vi "new_issue_full.vi"(11 "issueInfo":T1) -> (3 "issue_class out":refnum<class "issue_class.lvclass">)   [LabVIEW 2024, in "issue_class.lvclass"]
uses:
  issue_class.lvclass
  comic_class/issueInfo--cluster.ctl
  comic_class/creator--cluster.ctl
  comic_class/character--cluster.ctl
  comic_class/team--cluster.ctl
  comic_class/location--cluster.ctl
  comic_class/concept--cluster.ctl
  comic_class/thing--cluster.ctl
  comic_class/storyArc--cluster.ctl
  issue_class.lvclass/issue_class.ctl
  comic_class/comic_class.lvclass
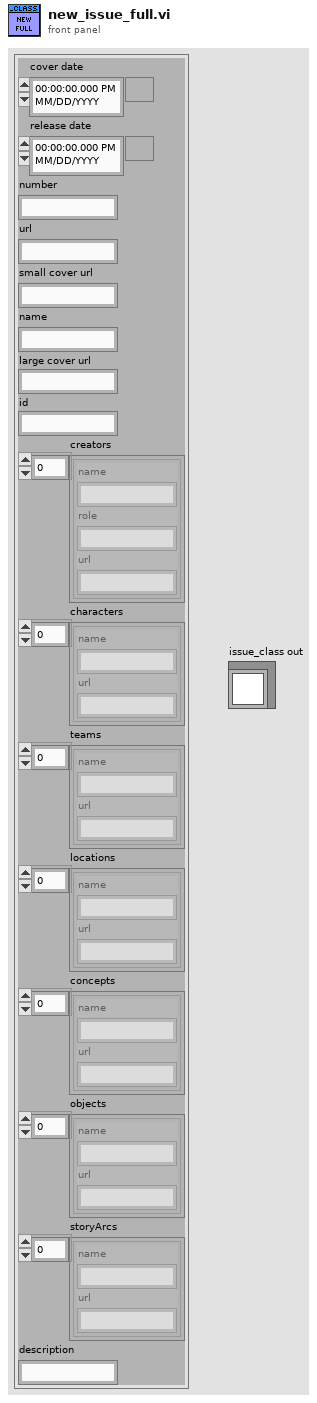
[diagram p1: front panel]
types:
  T1 = typedef "comic_class.lvclass/issueInfo--cluster.ctl" = cluster{"cover date":timestamp, "release date":timestamp, "number":string, "url":string, "small cover url":string, "name":string, "large cover url":string, "id":string, "creators":T2[], "characters":T3[], "teams":T4[], "locations":T5[], "concepts":T6[], "objects":T7[], "storyArcs":T8[], "description":string}
  T2 = typedef "comic_class.lvclass/creator--cluster.ctl" = cluster{"name":string, "role":string, "url":string}
  T3 = typedef "comic_class.lvclass/character--cluster.ctl" = cluster{"name":string, "url":string}
  T4 = typedef "comic_class.lvclass/team--cluster.ctl" = cluster{"name":string, "url":string}
  T5 = typedef "comic_class.lvclass/location--cluster.ctl" = cluster{"name":string, "url":string}
  T6 = typedef "comic_class.lvclass/concept--cluster.ctl" = cluster{"name":string, "url":string}
  T7 = typedef "comic_class.lvclass/thing--cluster.ctl" = cluster{"name":string, "url":string}
  T8 = typedef "comic_class.lvclass/storyArc--cluster.ctl" = cluster{"name":string, "url":string}
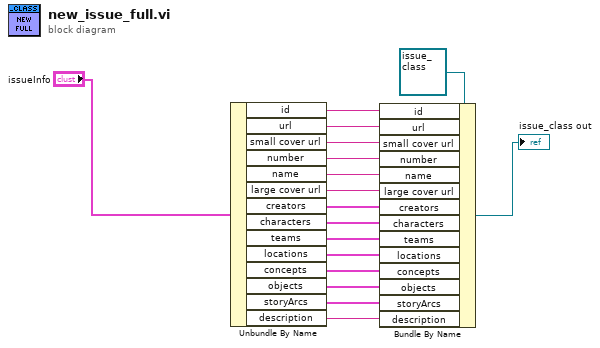
[diagram p0: block diagram]
diagram:
  n1 = Unbundle By Name("issueInfo") -> ("id"=w14:string, "url"=w13:string, "small cover url"=w12:string, "number"=w11:string, "name"=w10:string, "large cover url"=w9:string, "creators"=w8:T2[], "characters"=w7:T3[], "teams"=w6:T4[], "locations"=w5:T5[], "concepts"=w4:T6[], "objects"=w3:T7[], "storyArcs"=w2:T8[], "description"=w1:string)
  n2 = Bundle By Name(cluster=refnum<class "issue_class.lvclass"> refnum ("issue_class in"), "id"=w14, "url"=w13, "small cover url"=w12, "number"=w11, "name"=w10, "large cover url"=w9, "creators"=w8, "characters"=w7, "teams"=w6, "locations"=w5, "concepts"=w4, "objects"=w3, "storyArcs"=w2, "description"=w1) -> (→"issue_class out":refnum<class "issue_class.lvclass">)
